vi "download_udc_values.vi"(1 "Transfer Bar":refnum<vi>, 2 "UDC Table":string[][](array[string])) -> (0 "Value Array":dbl[](array[numeric]))   [LabVIEW 2011]
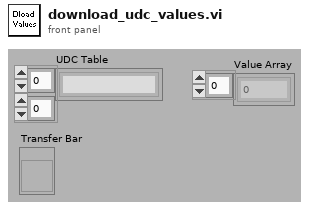
[diagram p1: front panel]
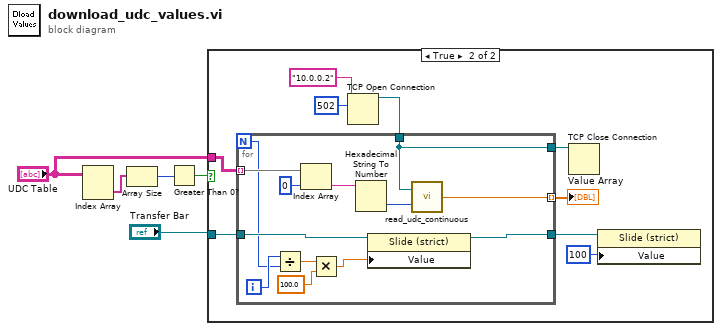
[diagram p0: block diagram]
diagram:
  n1 = Index Array(array="UDC Table") -> (element=w5:string[])  [unwired: 2 in]
  n2 = Array Size(array=w5) -> (size(s)=w1:i32)
  n3 = Greater Than 0?(x=w1) -> (x > 0?=w4:bool)
  n4 = case shown="True" w4 {
    tunnel: "UDC Table" -> [_ w11]
    tunnel: "Transfer Bar" -> [_ w10]
    frame False {
    }
    frame True {
      n5 = TCP Open Connection(address="10.0.0.2", remote port or service name=u16 502) -> (connection ID=w13:refnum<k5>)  [unwired: 1 in, 3 out]
      n6 = for {
        N -> [w16]
        tunnel: w11 -> [w27] mode=indexing
        tunnel: [w23] -> w14 mode=indexing
        tunnel: w13 -> [w22]
        tunnel: [w22] -> w12
        tunnel: w10 -> [w21]
        tunnel: [w15] -> w7
        i -> [w20]
        n7 = Divide(x=w20, y=w16) -> (x/y=w19:dbl)
        n8 = Index Array(array=w27, index=0) -> (element=w25:string)
        n9 = Multiply(x=w19, y=100.0) -> (x*y=w17:dbl)
        n10 = Hexadecimal String To Number(string=w25) -> (number=w24:u32)  [unwired: 3 out]
        n11 = property class="Slide (strict)"(reference=w21, "Value"=w17) -> (reference out=w15:refnum<vi>)  [unwired: 1 in, 1 out]
        n12 = call "read_udc_continuous.vi"("Hex Address"=w24, "TCP Connection Refnum in"=w22) -> ("Value"=w23:dbl)
      }
      "Value Array" <- w14
      n13 = TCP Close Connection(connection ID=w12) -> ()  [unwired: 1 in, 3 out]
      n14 = property class="Slide (strict)"(reference=w7, "Value"=u8 100) -> ()  [unwired: 1 in, 2 out]
    }
  }
